vi "MoveXYSteps.vi"(9 "Y Steps":dbl, 10 "X Steps":dbl) -> ()   [LabVIEW 2024]
uses:
  <vilib>/DAQmx/write.llb/DAQmx Write (Digital 1D Bool 1Chan 1Samp).vi
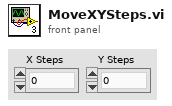
[diagram p1: front panel]
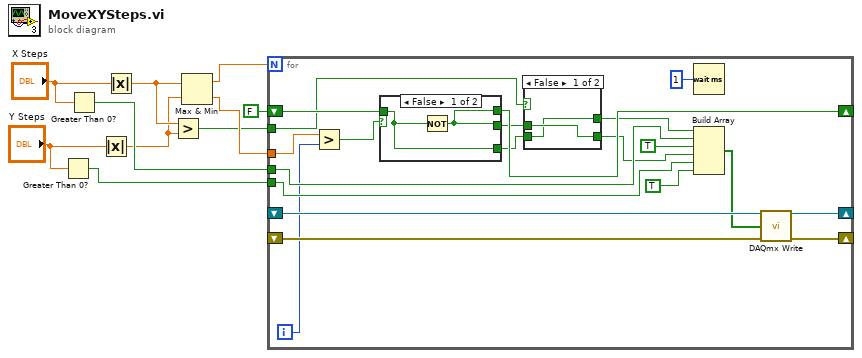
[diagram p0: block diagram]
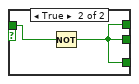
[diagram p3: hidden frame]
diagram:
  n1 = Greater Than 0?(x="Y Steps") -> (x > 0?=w7:bool)
  n2 = Greater Than 0?(x="X Steps") -> (x > 0?=w6:bool)
  n3 = Absolute Value(x="Y Steps") -> (abs(x)=w2:dbl)
  n4 = Absolute Value(x="X Steps") -> (abs(x)=w3:dbl)
  n5 = Greater?(x=w3, y=w2) -> (0:w1:bool)
  n6 = Max & Min(x=w3, y=w2) -> (max(x,y)=w5:dbl, min(x,y)=w4:dbl)
  n7 = for {
    N: w5 -> [_]
    shift-right: [w29] -> _
    shift-left: _ -> [w30]
    shift-right: [w27] -> _
    shift-left: _ -> [w28]
    shift-right: [w21] -> _
    shift-left: FALSE -> [w25]
    tunnel: w6 -> [w20]
    tunnel: w7 -> [w19]
    tunnel: w4 -> [w17]
    tunnel: w1 -> [w15]
    i -> [w18]
    n8 = Greater?(x=w17, y=w18) -> (0:w16:bool)
    n9 = case shown="False" w16 {
      tunnel: w25 -> [w36 w38]
      tunnel: [w35 w37] -> w21
      tunnel: [w36 w37] -> w14
      tunnel: [w35 w37] -> w13
      frame False {
        n10 = Not(x=w36) -> (.not. x?=w35:bool)
      }
      frame True {
        n11 = Not(x=w38) -> (.not. x?=w37:bool)
      }
    }
    n12 = case shown="False" w15 {
      tunnel: w14 -> [w31 w33]
      tunnel: w13 -> [w32 w34]
      tunnel: [w31 w34] -> w12
      tunnel: [w32 w33] -> w11
      frame False {
      }
      frame True {
      }
    }
    n13 = Wait (ms)(milliseconds to wait=u32 1) -> ()  [unwired: 1 out]
    n14 = Build Array(w12, w20, TRUE, w11, w19, TRUE) -> (w23:bool[])
    n15 = call-poly <vilib>:"DAQmx Write.vi"("task/channels in"=w30, "data"=w23, "error in"=w28) -> ("task out"=w29:refnum<k21>, "error out"=w27:errorcluster)  [unwired: 10 in, 1 out]
  }
